vi "FestoCPX.Station.ProdPresent.Wait.vi"(5 "AllowSingleSlot":bool, 7 "SuckerID (0: Final)":i32, 8 "error in":errorcluster) -> (0 "error out":errorcluster, 3 "Present.SuckerID":cluster{"A":bool, "B":bool})   [LabVIEW 2016]
uses:
  Station/Station.ValvePosition.ctl
  Station/Station.ProductSlot.ctl
panel:
  out "Debug":cluster{"A":bool, "B":bool}
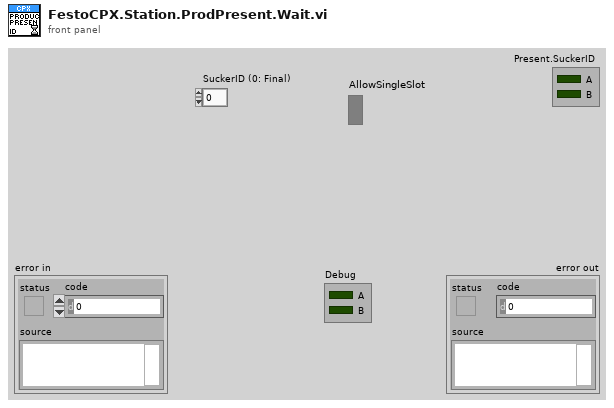
[diagram p1: front panel]
types:
  T1 = typedef "Station.ProductSlot.ctl" = enum8{"A", "B"}
  T2 = typedef "FestoCPX.Station.ProdPresent.ctl" = cluster{"Slot1":cluster{"A":bool, "B":bool}, "Slot2":cluster{"A":bool, "B":bool}, "Slot3":cluster{"A":bool, "B":bool}, "Slot4":cluster{"A":bool, "B":bool}, "Final":cluster{"A":bool, "B":bool}, "OK":cluster{"A":bool, "B":bool}, "Container":cluster{"OK":bool, "NOK":bool}}
  T3 = typedef "Station.ValvePosition.ctl" = enum16{"Home", "Work"}
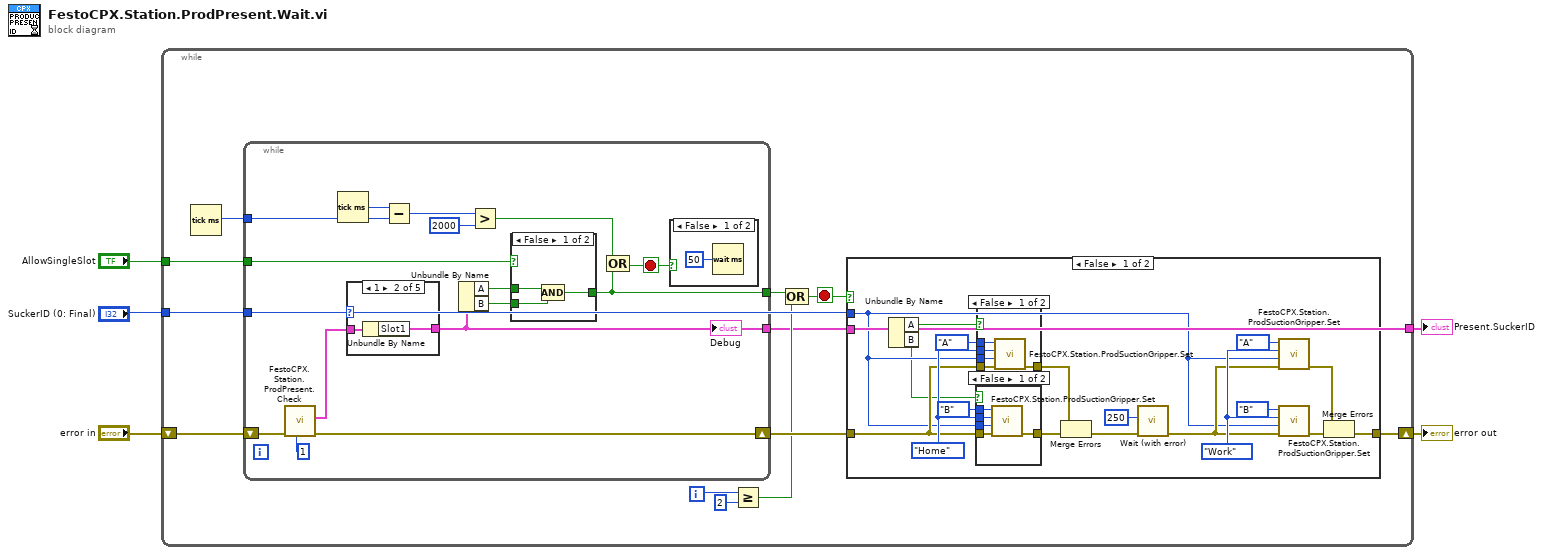
[diagram p0: block diagram]
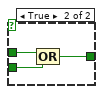
[diagram p5: hidden frame]
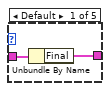
[diagram p7: hidden frame]
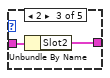
[diagram p8: hidden frame]
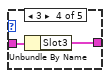
[diagram p9: hidden frame]
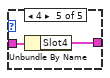
[diagram p10: hidden frame]
diagram:
  n1 = while {
    tunnel: "SuckerID (0: Final)" -> [w12]
    tunnel: [w6] -> w2
    tunnel: "AllowSingleSlot" -> [w15]
    shift-right: [w11] -> w3
    shift-left: "error in" -> [w17]
    i -> [w10]
    stop <- w7 stop-if-true
    n2 = Tick Count (ms)() -> (millisecond timer value=w16:u32)
    n3 = while {
      tunnel: w12 -> [w65]
      tunnel: [w52] -> w6
      shift-right: [w63] -> w13
      shift-left: w17 -> [w64]
      tunnel: w16 -> [w58]
      tunnel: w15 -> [w53]
      tunnel: [w51] -> w14
      stop <- w54 stop-if-true
      n4 = call "FestoCPX.Station.ProdPresent.Check.vi"("Stab Counter (0)"=1 ("Max Stab time [ms] (0)"), "error in"=w64) -> ("error out"=w63:errorcluster, "Prod Present"=w62:T2)  [unwired: 4 in, 4 out]
      n5 = Tick Count (ms)() -> (millisecond timer value=w59:u32)
      n6 = case shown="1" w65 {
        tunnel: w62 -> [w74 w76 w78 w80 w82]
        tunnel: [w73 w75 w77 w79 w81] -> w52
        frame Default {
          n7 = Unbundle By Name(w74) -> ("Final"=w73:cluster{"A":bool, "B":bool})
        }
        frame 1 {
          n8 = Unbundle By Name(w76) -> ("Slot1"=w75:cluster{"A":bool, "B":bool})
        }
        frame 2 {
          n9 = Unbundle By Name(w78) -> ("Slot2"=w77:cluster{"A":bool, "B":bool})
        }
        frame 3 {
          n10 = Unbundle By Name(w80) -> ("Slot3"=w79:cluster{"A":bool, "B":bool})
        }
        frame 4 {
          n11 = Unbundle By Name(w82) -> ("Slot4"=w81:cluster{"A":bool, "B":bool})
        }
      }
      "Debug" <- w52
      n12 = Subtract(x=w59, y=w58) -> (x-y=w57:u32)
      n13 = Unbundle By Name(w52) -> ("A"=w61:bool, "B"=w60:bool)
      n14 = Greater?(x=w57, y=u32 2000) -> (0:w55:bool)
      n15 = case shown="False" w53 {
        tunnel: w61 -> [w68 w71]
        tunnel: w60 -> [w67 w70]
        tunnel: [w66 w69] -> w51
        frame False {
          n16 = Compound Arithmetic op=AND(w68, w67) -> (w66:bool)
        }
        frame True {
          n17 = Compound Arithmetic op=OR(w71, w70) -> (w69:bool)
        }
      }
      n18 = Compound Arithmetic op=OR(w55, w51) -> (w54:bool)
      n19 = case shown="False" w54 {
        frame False {
          n20 = Wait (ms)(milliseconds to wait=u32 50) -> ()  [unwired: 1 out]
        }
        frame True {
        }
      }
    }
    n21 = Greater Or Equal?(x=w10, y=2) -> (x >= y?=w8:bool)
    n22 = Compound Arithmetic op=OR(w14, w8) -> (w7:bool)
    n23 = case shown="False" w7 {
      tunnel: w13 -> [w33 w49]
      tunnel: w12 -> [w21 _]
      tunnel: [w22 w49] -> w11
      tunnel: w6 -> [w20 _]
      frame False {
        w30 = Station.ValvePosition."Work" ("Position")
        w34 = Station.ValvePosition."Home" ("Position")
        n24 = Unbundle By Name(w20) -> ("A"=w19:bool, "B"=w18:bool)
        n25 = case shown="False" w18 {
          tunnel: Station.ProductSlot."B" ("Slot") -> [w41 _]
          tunnel: w34 -> [w40 _]
          tunnel: w33 -> [w39 w42]
          tunnel: [w38 w42] -> w29
          tunnel: w21 -> [w37 _]
          frame False {
            n26 = call "FestoCPX.Station.ProdSuctionGripper.Set.vi"("error in"=w39, "Sucker (0: Final)"=w37, "Position"=w40, "Slot"=w41) -> ("error out"=w38:errorcluster)  [unwired: 6 in, 1 out]
          }
          frame True {
          }
        }
        n27 = case shown="False" w19 {
          tunnel: Station.ProductSlot."A" ("Slot") -> [w47 _]
          tunnel: w34 -> [w46 _]
          tunnel: w33 -> [w45 w48]
          tunnel: [w44 w48] -> w28
          tunnel: w21 -> [w43 _]
          frame False {
            n28 = call "FestoCPX.Station.ProdSuctionGripper.Set.vi"("error in"=w45, "Sucker (0: Final)"=w43, "Position"=w46, "Slot"=w47) -> ("error out"=w44:errorcluster)  [unwired: 6 in, 1 out]
          }
          frame True {
          }
        }
        n29 = Merge Errors(w28, w29) -> (w23:errorcluster)
        n30 = call "Wait (with error).vi"("error in (no error)"=w23, "milliseconds to wait"=u32 250) -> ("error out"=w24:errorcluster)  [unwired: 8 in, 1 out]
        n31 = call "FestoCPX.Station.ProdSuctionGripper.Set.vi"("error in"=w24, "Sucker (0: Final)"=w21, "Position"=w30, "Slot"=Station.ProductSlot."A") -> ("error out"=w26:errorcluster)  [unwired: 6 in, 1 out]
        n32 = call "FestoCPX.Station.ProdSuctionGripper.Set.vi"("error in"=w24, "Sucker (0: Final)"=w21, "Position"=w30, "Slot"=Station.ProductSlot."B") -> ("error out"=w27:errorcluster)  [unwired: 6 in, 1 out]
        n33 = Merge Errors(w26, w27) -> (w22:errorcluster)
      }
      frame True {
      }
    }
  }
  "error out" <- w3
  "Present.SuckerID" <- w2
